vi "Remove Data Point.vi"(8 "pixel position":cluster{"X":i32, "Y":i32}, 9 "DrawAreaSize":T1={"Width"=100, "Height"=100}, 10 "draw options":T2={"Background Color"=16777215, "Grid Color"=13816530, "Angle Units"=enum."Degrees", "Draw Solid Background"=TRUE, "Draw Grid"=TRUE, "Grid Spacing"=0.25, "AutoScale"=FALSE, "Fit to Radius"=1.0, "data row options"=[]}, 11 "data in":T5) -> (3 "data out":T5)   [LabVIEW 2017, in "NI_Robotics_2D Rangefinder Picture.lvlib"]
uses:
  <vilib>/robotics/Controls/2D Rangefinder/2D Rangefinder Picture/NI_Robotics_2D Rangefinder Picture.lvlib
  <vilib>/robotics/Controls/2D Rangefinder/2D Rangefinder Picture/Rangefinder Data.ctl
  <vilib>/robotics/Controls/2D Rangefinder/2D Rangefinder Picture/Draw Options.ctl
  <vilib>/robotics/Controls/Utilities/Angle Units.ctl
  <vilib>/robotics/Controls/2D Rangefinder/2D Rangefinder Picture/Data Row Options.ctl
  <vilib>/Utility/miscctls.llb/LVBoundsTypeDef.ctl
  <vilib>/Utility/AngleManip/Degrees to Radians.vi
  <vilib>/Utility/AngleManip/Degrees to Radians (Array DBL).vi
  <vilib>/robotics/Controls/Utilities/NI_Robotics_Control Utilities.lvlib
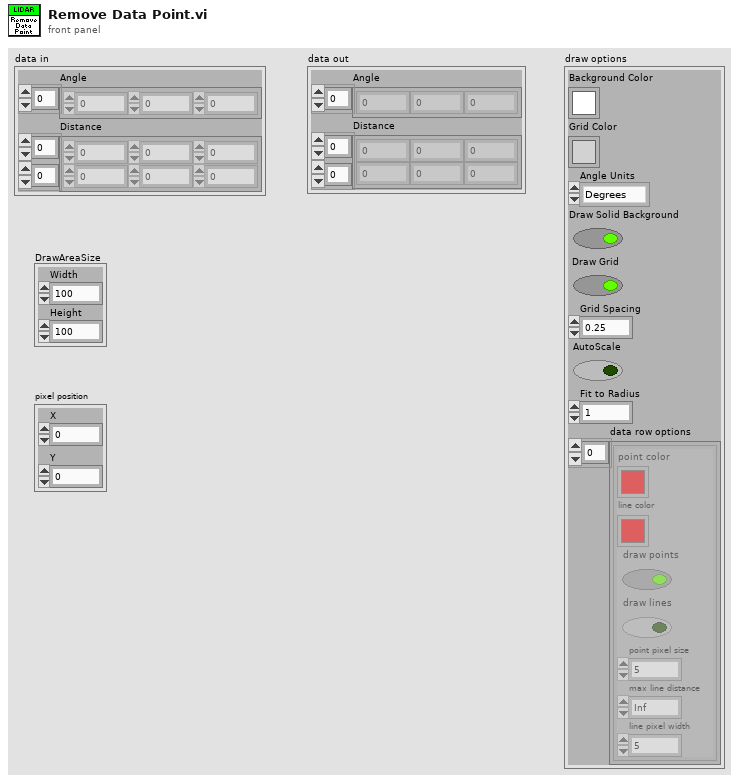
[diagram p1: front panel]
types:
  T1 = typedef "LVBoundsTypeDef.ctl" = cluster{"Width":u32, "Height":u32}
  T2 = typedef "NI_Robotics_2D Rangefinder Picture.lvlib/Draw Options.ctl" = cluster{"Background Color":u32, "Grid Color":u32, "Angle Units":T3, "Draw Solid Background":bool, "Draw Grid":bool, "Grid Spacing":dbl, "AutoScale":bool, "Fit to Radius":dbl, "data row options":T4[]}
  T3 = typedef "NI_Robotics_Control Utilities.lvlib/Angle Units.ctl" = enum16{"Radians", "Degrees"}
  T4 = typedef "NI_Robotics_2D Rangefinder Picture.lvlib/Data Row Options.ctl" = cluster{"point color":u32, "line color":u32, "draw points":bool, "draw lines":bool, "point pixel size":u16, "max line distance":dbl, "line pixel width":u16}
  T5 = typedef "NI_Robotics_2D Rangefinder Picture.lvlib/Rangefinder Data.ctl" = cluster{"Angle":dbl[], "Distance":dbl[][]}
  T6 = typedef "NI_Robotics_2D Rangefinder Picture.lvlib/Cartesian Data.ctl" = cluster{"xy points":cluster{"xy set":cluster{"x":dbl, "y":dbl}[], "distance set":dbl[]}[], "max radius":dbl}
  T7 = typedef "NI_Robotics_2D Rangefinder Picture.lvlib/Scaling Info.ctl" = cluster{"pixels per unit":dbl, "fit radius (units)":dbl, "center point (pixels)":cluster{"x":i16, "y":i16}}
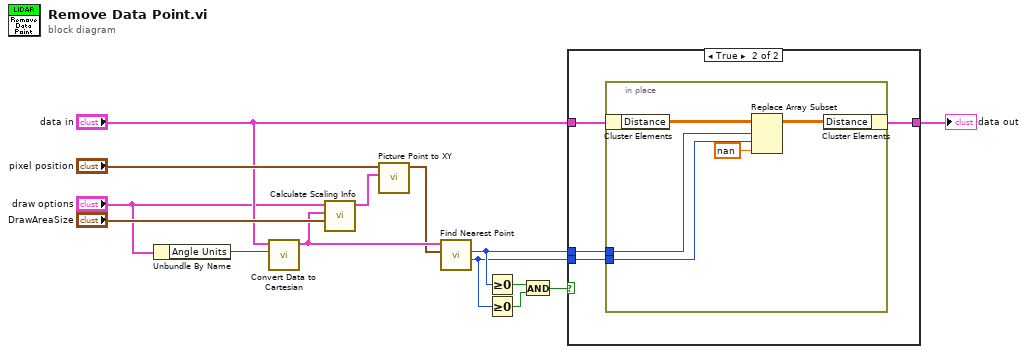
[diagram p0: block diagram]
diagram:
  n1 = Unbundle By Name("draw options") -> ("Angle Units"=w8:T3)
  n2 = call <vilib>:"Convert Data to Cartesian.vi"("angle units"=w8, "data"="data in") -> ("cartesian data"=w7:T6)  [unwired: 9 in]
  n3 = call <vilib>:"Calculate Scaling Info.vi"("DrawAreaSize"="DrawAreaSize", "cartesian data"=w7, "draw options in"="draw options") -> ("scaling info"=w12:T7)  [unwired: 8 in]
  n4 = call <vilib>:"Picture Point to XY.vi"("scaling info"=w12, "xy point (pixels)"="pixel position") -> ("xy point (units)"=w6:cluster{"x":dbl, "y":dbl})  [unwired: 9 in]
  n5 = call <vilib>:"Find Nearest Point.vi"("xy point (units)"=w6, "cartesian data"=w7) -> ("col"=w1:i32, "row"=w2:i32)  [unwired: 7 in, 1 out]
  n6 = Greater Or Equal To 0?(x=w2) -> (x >= 0?=w5:bool)
  n7 = Greater Or Equal To 0?(x=w1) -> (x >= 0?=w4:bool)
  n8 = And(x=w5, y=w4) -> (x .and. y?=w3:bool)
  n9 = case shown="True" w3 {
    tunnel: "data in" -> [w15 w19]
    tunnel: [w15 w18] -> w10
    tunnel: w2 -> [_ w17]
    tunnel: w1 -> [_ w16]
    frame False {
    }
    frame True {
      n10 = in-place {
        in-place-border: w17 -> [w22]
        in-place-border: w16 -> [w21]
        n11 = in-place-cluster #1(w19) -> ("Distance"=w24:dbl[][])
        n12 = Replace Array Subset(array=w24, new element=nan ("new element/subarray"), index (row)=w22, index (col)=w21) -> (w23:dbl[][])
        n13 = in-place-cluster #1("Distance"=w23) -> (w18:T5)
      }
    }
  }
  "data out" <- w10
